vi "Write Folder Shot File.vi"(8 "error in (no error)":errorcluster, 10 "Folder Shot":T1[](array[typedef]), 11 "Log Path":path) -> (0 "error out":errorcluster)   [LabVIEW 2016, in "SLL File IO.lvlib"]
doc: "Writes the Folder Shot Cluster Array to File."
uses:
  SLL File IO.lvlib
  _Typedefs/Folder Shot Element.ctl
  <vilib>/Utility/file.llb/Write Delimited Spreadsheet (string).vi
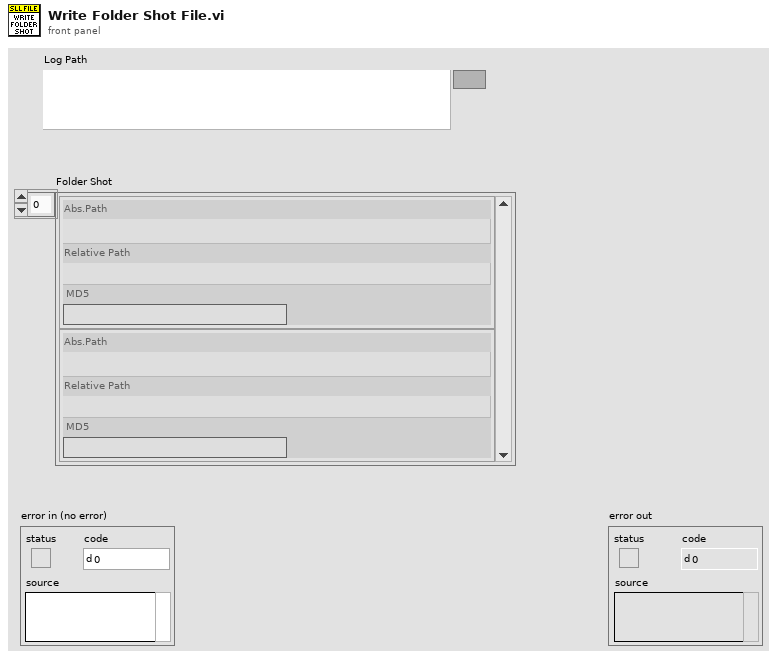
[diagram p1: front panel]
types:
  T1 = typedef "SLL File IO.lvlib/Folder Shot Element.ctl" = cluster{"Abs.Path":path, "Relative Path":path, "MD5":string}
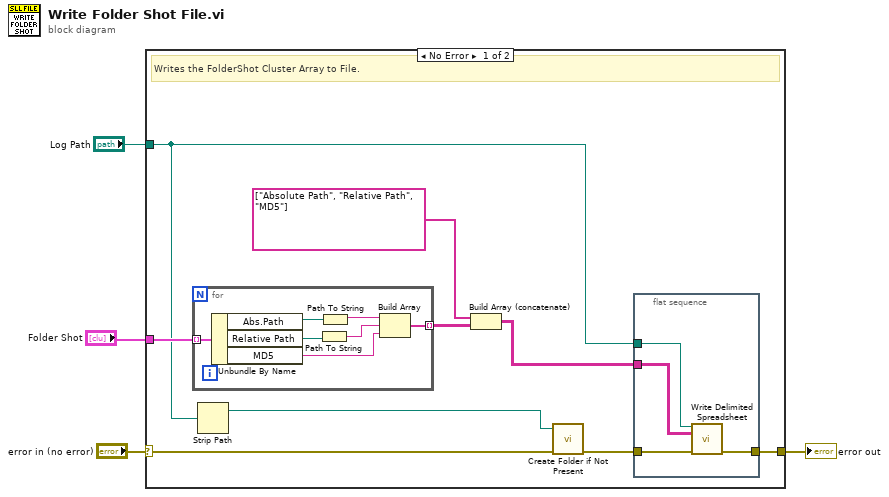
[diagram p0: block diagram]
diagram:
  n1 = case shown="No Error" "error in (no error)" {
    selector: "error in (no error)" -> [w9 w25]
    tunnel: [w7 w25] -> w3
    tunnel: "Log Path" -> [w6 _]
    tunnel: "Folder Shot" -> [w13 _]
    frame No Error {
      # "Writes the FolderShot Cluster Array to File."
      n2 = for {
        tunnel: w13 -> [w24] mode=indexing
        tunnel: [w18] -> w11 mode=indexing
        n3 = Unbundle By Name(w24) -> ("Abs.Path"=w23:path, "Relative Path"=w22:path, "MD5"=w19:string)
        n4 = Path To String(path=w22) -> (string=w20:string)
        n5 = Path To String(path=w23) -> (string=w21:string)
        n6 = Build Array(w21, w20, w19) -> (w18:string[])
      }
      n7 = Strip Path(path=w6) -> (stripped path=w5:path)  [unwired: 1 out]
      n8 = Build Array (concatenate)(string[] ["Absolute Path", "Relative Path", "MD5"], w11) -> (w10:string[][])
      n9 = call "Create Folder if Not Present.vi"("error in (no error)"=w9, "Path"=w5) -> ("error out"=w8:errorcluster)  [unwired: 8 in, 1 out]
      n10 = flat-sequence {
        tunnel: w6 -> [w17]
        tunnel: w10 -> [w16]
        tunnel: w8 -> [w15]
        tunnel: [w14] -> w7
        frame #0 {
          n11 = call-poly <vilib>:"Write Delimited Spreadsheet.vi"("file path (dialog if empty)"=w17, "2D data"=w16, "error in (no error)"=w15) -> ("error out"=w14:errorcluster)  [unwired: 11 in, 1 out]
        }
      }
    }
    frame Error {
    }
  }
  "error out" <- w3
